vi "Panel.vi"(8 "error in (no error)":errorcluster, 11 "Rate Step in":refnum<class "Rate Step.lvclass">) -> ()   [LabVIEW 2018, in "Temp Recipe.lvlib" / "Rate Step.lvclass"]
uses:
  Rate Step.lvclass
  C:/dev/source/Systems/NI Week/Temperature Recipe/Temp Recipe/Recipe Step/Recipe Step.lvclass
  C:/dev/source/Libraries/OOPanel/OOPanel/Panel/Panel.lvclass
  Libraries/OOPanel/OOPanel/Panel/Panel.lvclass
  Libraries/OOPanel/OOPanel/PanelArray/PanelArray.lvclass
  Recipe Step/Recipe Step.lvclass
panel:
  in  "Target":dbl format="%.1f °F"
  in  "Remove Button":bool
  in  "Down Button":bool
  in  "Up Button":bool
  in  "Step Time":dbl format="%.0f Minutes"
  in  "Step Temp":dbl format="%.1f °F"
  # "per"
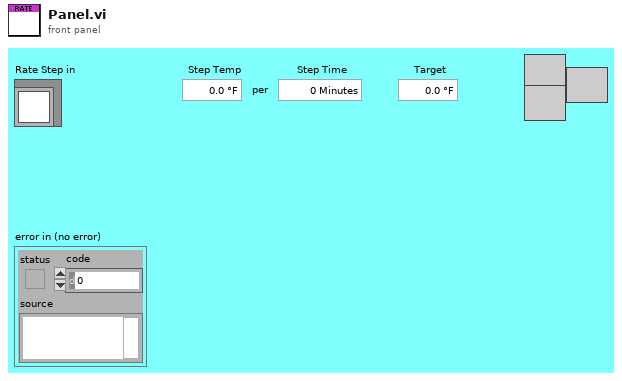
[diagram p1: front panel]
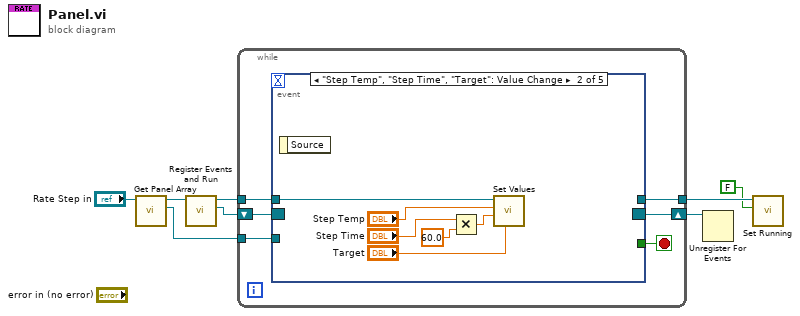
[diagram p0: block diagram]
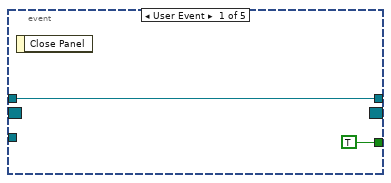
[diagram p2: hidden frame]
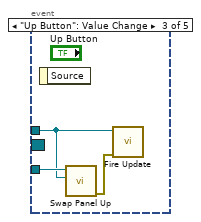
[diagram p3: hidden frame]
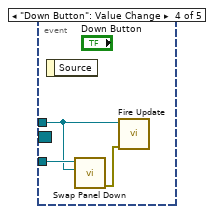
[diagram p4: hidden frame]
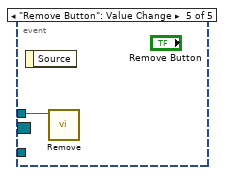
[diagram p5: hidden frame]
diagram:
  n1 = call "Get Panel Array.vi"("Recipe Step in"="Rate Step in") -> ("PanelArray"=w1:refnum<class "PanelArray.lvclass">, "Recipe Step out"=w2:refnum<class "Rate Step.lvclass">)  [unwired: 8 in, 1 out]
  n2 = call "Register Events and Run.vi"("Panel in"=w2) -> ("Event Registration Refnum"=w7:refnum<event-registration>, "Panel out"=w8:refnum<class "Rate Step.lvclass">)  [unwired: 8 in, 1 out]
  n3 = while {
    tunnel: w8 -> [w13]
    shift-right: [w11] -> w6
    shift-left: w7 -> [w14]
    tunnel: [w10] -> w5
    tunnel: w1 -> [w9]
    stop <- w12 stop-if-true
    n4 = event shown="[1] \"Step Temp\", \"Step Time\", \"Target\": Value Change" {
      selector: w14 -> [_ _ _ _ _]
      dyn-events: [_ _ _ _ _] -> w11
      timeout: _ -> [_ _ _ _ _]
      tunnel: w13 -> [w15 w22 w24 w27 w29]
      tunnel: [TRUE _ _ _ _] -> w12
      tunnel: [w15 _ _ _ _] -> w10
      tunnel: w9 -> [_ _ w25 w28 _]
      event User Event {
        n5 = event-data() -> ()  [unwired: 1 in, 1 out]
      }
      event "Step Temp", "Step Time", "Target": Value Change {
        n6 = event-data() -> ()  [unwired: 1 in, 1 out]
        n7 = Multiply(x="Step Time", y=60.0) -> (x*y=w19:dbl)
        n8 = call "Set Values.vi"("Target"="Target", "Step Time"=w19, "Step Temp"="Step Temp", "Rate Step in"=w22) -> ()  [unwired: 6 in, 2 out]
      }
      event "Up Button": Value Change {
        n9 = event-data() -> ()  [unwired: 1 in, 1 out]
        n10 = call "Swap Panel Up.vi"("Panel"=w24, "PanelArray in"=w25) -> ("error out"=w23:errorcluster)  [unwired: 8 in, 1 out]
        n11 = call "Fire Update.vi"("error in (no error)"=w23, "Recipe Step in"=w24) -> ()  [unwired: 8 in, 2 out]
      }
      event "Down Button": Value Change {
        n12 = event-data() -> ()  [unwired: 1 in, 1 out]
        n13 = call "Swap Panel Down.vi"("Panel"=w27, "PanelArray in"=w28) -> ("error out"=w26:errorcluster)  [unwired: 8 in, 1 out]
        n14 = call "Fire Update.vi"("error in (no error)"=w26, "Recipe Step in"=w27) -> ()  [unwired: 8 in, 2 out]
      }
      event "Remove Button": Value Change {
        n15 = event-data() -> ()  [unwired: 1 in, 1 out]
        n16 = call "Remove.vi"("Recipe Step in"=w29) -> ()  [unwired: 9 in, 2 out]
      }
    }
  }
  n17 = Unregister For Events(event registration refnum=w6) -> ()  [unwired: 1 in, 1 out]
  n18 = call "Set Running.vi"("Running"=FALSE, "Panel in"=w5) -> ()  [unwired: 8 in, 2 out]
